vi "原点回归设置.vi"() -> (0 "LastPra out":T1, 3 "ok":bool)   [LabVIEW 2011]
panel:
  in  "LastPra":T1
  in  "取消按钮":bool
  in  "确定按钮":bool
  in  "Y轴原点回归爬行速度":u32
  in  "X轴原点回归爬行速度":u32
  in  "Y轴原点回归速度":u32
  in  "X轴原点回归速度":u32
  # "X轴原点参数设置"
  # "Y轴原点参数设置"
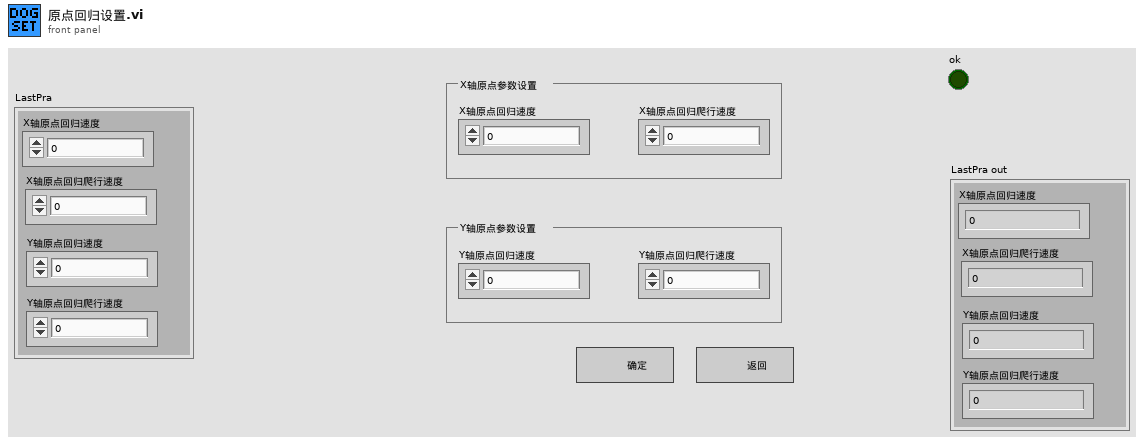
[diagram p1: front panel]
types:
  T1 = typedef "DOG参数.ctl" = cluster{"X轴原点回归速度":u32, "X轴原点回归爬行速度":u32, "Y轴原点回归速度":u32, "Y轴原点回归爬行速度":u32}
  T2 = enum16{"open", "replace", "create", "open or create", "replace or create", "replace or create with confirmation"}
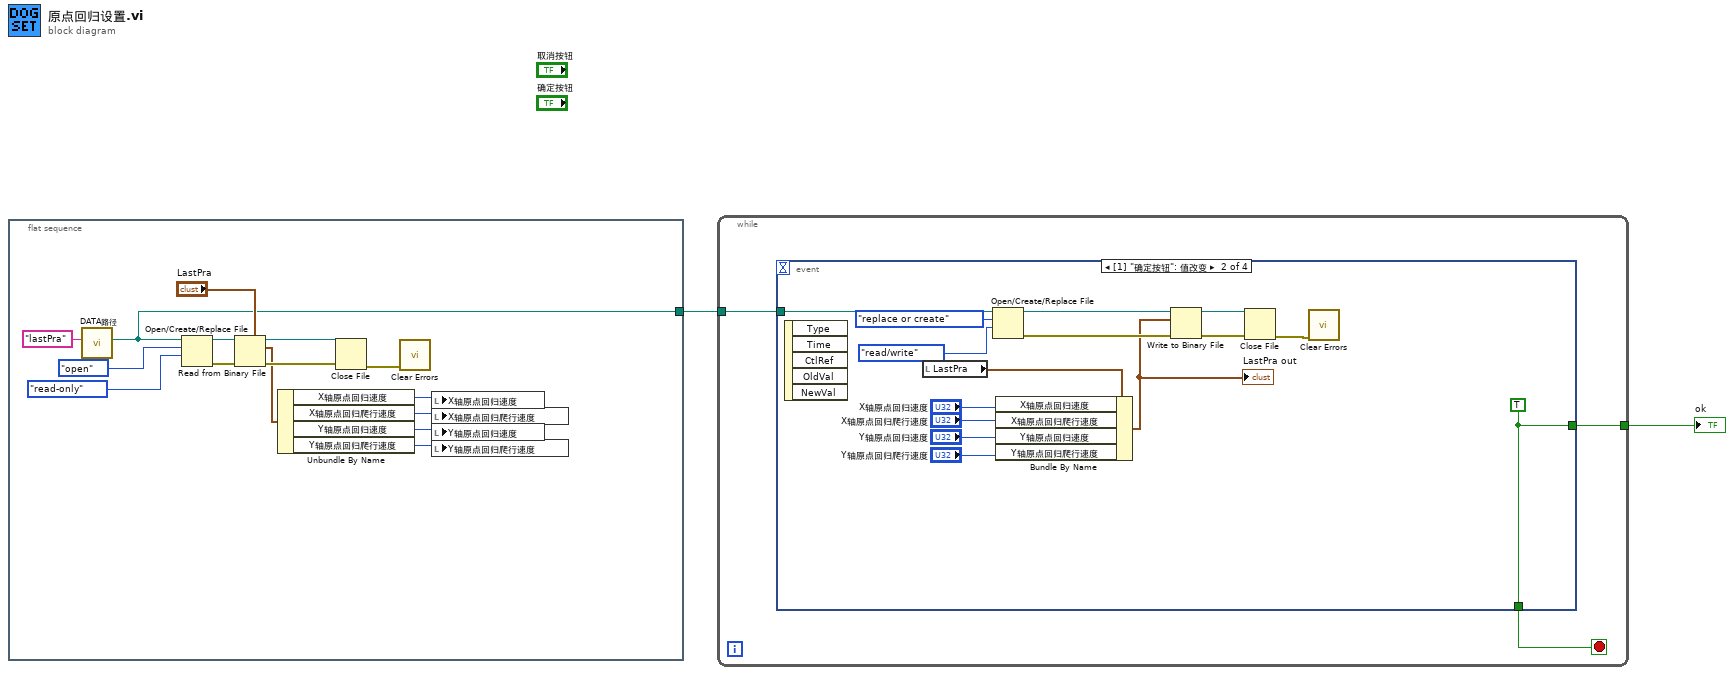
[diagram p0: block diagram]
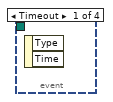
[diagram p2: hidden frame]
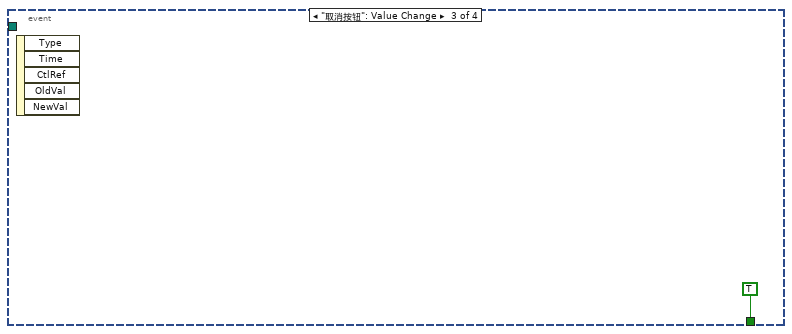
[diagram p3: hidden frame]
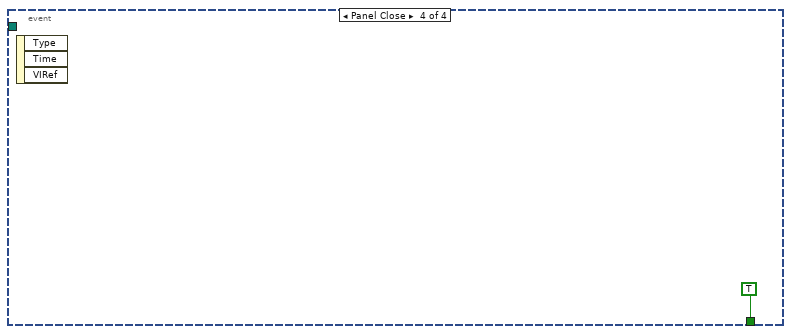
[diagram p4: hidden frame]
diagram:
  n1 = flat-sequence {
    tunnel: [w3] -> w2
    frame #0 {
      n2 = call "DATA路径.vi"("文件名"="lastPra") -> ("DATA路径"=w3:path)  [unwired: 10 in]
      n3 = Open/Create/Replace File(file path (use dialog)=w3, operation (0:open)=T2."open" ("操作(0:open)"), access (0:read/write)=enum16{"read/write", "read-only", "write-only"}."read-only" ("权限(0:read/write)")) -> (refnum out=w14:refnum<file>, error out=w13:errorcluster)  [unwired: 3 in, 1 out]
      n4 = Read from Binary File(5:"LastPra", 8:w13, 11:w14) -> (0:w11:errorcluster, 2:w8:T1, 3:w12:refnum<file>)  [unwired: 3 in, 1 out]
      n5 = Unbundle By Name(w8) -> ("X轴原点回归速度"=w7:u32, "X轴原点回归爬行速度"=w6:u32, "Y轴原点回归速度"=w5:u32, "Y轴原点回归爬行速度"=w4:u32)
      n6 = Close File(refnum=w12, error in=w11) -> (error out=w10:errorcluster)  [unwired: 1 out]
      n7 = call <vilib>:"Clear Errors.vi"("error in (no error)"=w10) -> ()  [unwired: 6 in, 1 out]
      n8 = local write "X轴原点回归速度"(w7) -> ()
      n9 = local write "X轴原点回归爬行速度"(w6) -> ()
      n10 = local write "Y轴原点回归速度"(w5) -> ()
      n11 = local write "Y轴原点回归爬行速度"(w4) -> ()
    }
  }
  n12 = while {
    tunnel: w2 -> [w19]
    tunnel: [w18] -> w1
    stop <- w20 stop-if-true
    n13 = event shown="[1] \"确定按钮\": 值改变" {
      selector: _ -> [_ _ _ _]
      dyn-events: _ -> [_ _ _ _]
      timeout: _ -> [_ _ _ _]
      tunnel: [_ w21 TRUE TRUE] -> w20
      tunnel: w19 -> [_ w35 _ _]
      tunnel: [_ w21 _ _] -> w18
      event Timeout {
        n14 = event-data() -> ()  [unwired: 1 in, 2 out]
      }
      event "确定按钮": Value Change {
        w21 = TRUE
        n15 = event-data() -> ()  [unwired: 1 in, 5 out]
        n16 = local read "LastPra"() -> (w30:T1)
        n17 = Open/Create/Replace File(file path (use dialog)=w35, operation (0:open)=T2."replace or create" ("操作(0:open)"), access (0:read/write)=enum16{"read/write", "read-only", "write-only"}."read/write" ("权限(0:read/write)")) -> (refnum out=w32:refnum<file>, error out=w31:errorcluster)  [unwired: 3 in, 1 out]
        n18 = Bundle By Name(cluster=w30, "X轴原点回归速度"="X轴原点回归速度", "X轴原点回归爬行速度"="X轴原点回归爬行速度", "Y轴原点回归速度"="Y轴原点回归速度", "Y轴原点回归爬行速度"="Y轴原点回归爬行速度") -> (w22:T1)
        "LastPra out" <- w22
        n19 = Write to Binary File(file (use dialog)=w32, data=w22, error in=w31) -> (refnum out=w25:refnum<file>, error out=w24:errorcluster)  [unwired: 3 in, 1 out]
        n20 = Close File(refnum=w25, error in=w24) -> (error out=w23:errorcluster)  [unwired: 1 out]
        n21 = call <vilib>:"Clear Errors.vi"("error in (no error)"=w23) -> ()  [unwired: 6 in, 1 out]
      }
      event "取消按钮": Value Change {
        n22 = event-data() -> ()  [unwired: 1 in, 5 out]
      }
      event Panel Close {
        n23 = event-data() -> ()  [unwired: 1 in, 3 out]
      }
    }
  }
  "ok" <- w1
